vi "TemplateVI.vi"(8 "error in (no error)":errorcluster, 11 "CCD in":refnum<class "CCD.lvclass">) -> (0 "error out":errorcluster, 3 "CCD out":refnum<class "CCD.lvclass">)   [LabVIEW 2023, in "CCD.lvclass"]
uses:
  CCD.lvclass
  CCD.lvclass/CCD.ctl
  20f7d3bd-08ac-4524-9bed-df36c1da25a0.vi
  a21955fc-e3a0-4e36-8495-41f1bfac7860.vi
  GenericDevice/GenericDevice.lvclass
panel:
  # "Connector Pane"
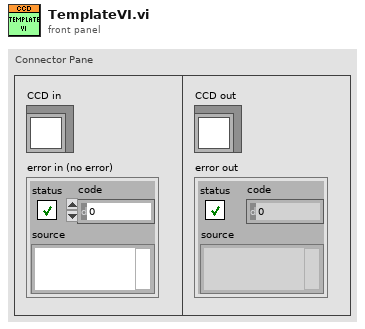
[diagram p1: front panel]
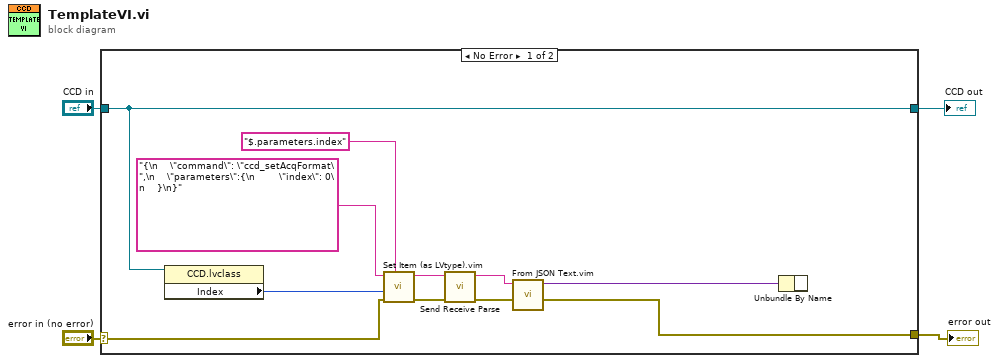
[diagram p0: block diagram]
diagram:
  n1 = case shown="No Error" "error in (no error)" {
    selector: "error in (no error)" -> [w11 w17]
    tunnel: [w10 w17] -> w3
    tunnel: [w13 w16] -> w1
    tunnel: "CCD in" -> [w13 w16]
    frame No Error {
      n2 = property class="CCD.lvclass"(reference=w13) -> ("Index"=w12:i32)  [unwired: 1 in, 2 out]
      n3 = call "Set Item (as LVtype).vim"("$Path or Item Name"="$.parameters.index", "error in (no error)"=w11, "Anything"=w12, "JSON"="{\n    \"command\": \"ccd_setAcqFormat\",\n    \"parameters\":{\n        \"index\": 0\n    }\n}") -> ("error out"=w7:errorcluster, "<JSON>"=w9:string)  [unwired: 4 in, 1 out]
      n4 = call "Send Receive Parse.vi"("error in"=w7, "<JSON>"=w9) -> ("error out"=w6:errorcluster, "results-JSON string"=w8:string)  [unwired: 7 in, 1 out]
      n5 = call "From JSON Text.vim"("error in (no error)"=w6, "JSON"=w8) -> ("error out"=w10:errorcluster, "Data out"=w5:variant)  [unwired: 8 in]
      n6 = Unbundle By Name(w5) -> ()  [unwired: 1 out]
    }
    frame Error {
    }
  }
  "error out" <- w3
  "CCD out" <- w1
